vi "Write ITX.vi"(6 "Commands":string, 8 "error in":errorcluster, 9 "Notes":string, 10 "Data (Dictionary)":T1[](array[typedef]), 11 "filename":path) -> (0 "error out":errorcluster, 3 "file":path)   [LabVIEW 2020, in "Data.ITX.lvclass"]
uses:
  Data.ITX.lvclass
  Data/Typedefs/Dictionary--cluster.ctl
  Data/Data.lvclass
panel:
  out "String":string
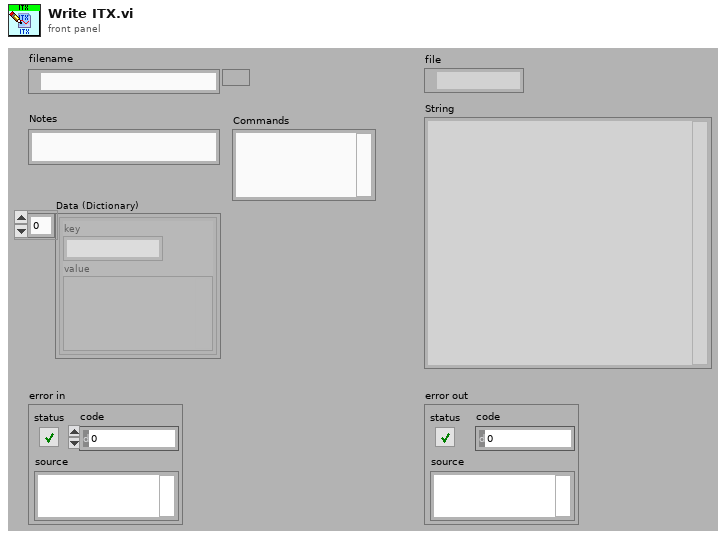
[diagram p1: front panel]
types:
  T1 = typedef "Data.lvclass/Dictionary--cluster.ctl" = cluster{"key":string, "value":variant}
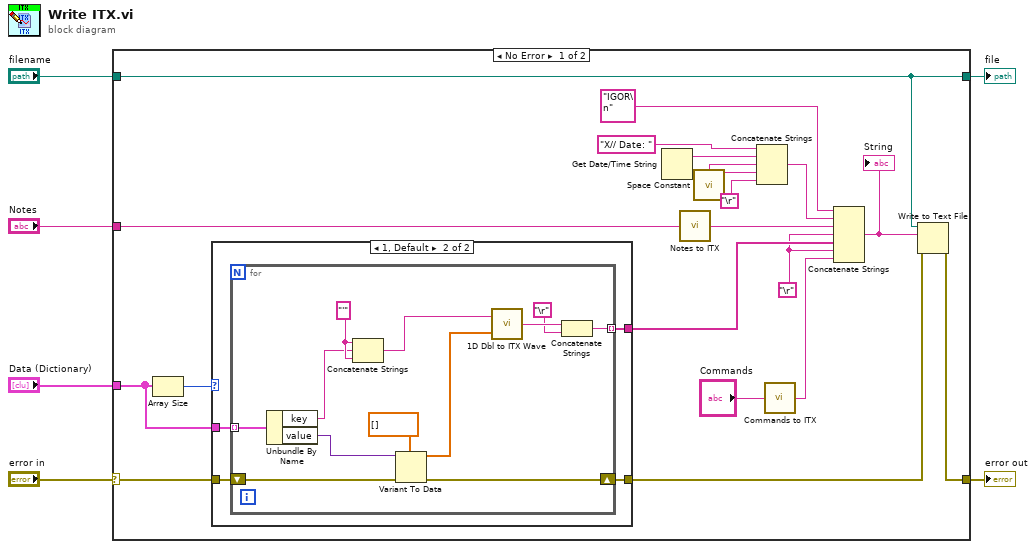
[diagram p0: block diagram]
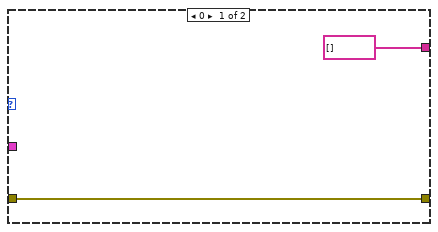
[diagram p2: hidden frame]
diagram:
  n1 = case shown="No Error" "error in" {
    selector: "error in" -> [w8 w45]
    tunnel: "filename" -> [w9 w46]
    tunnel: "Notes" -> [w19 _]
    tunnel: [w13 w45] -> w4
    tunnel: "Data (Dictionary)" -> [w10 _]
    tunnel: [w9 w46] -> w2
    frame No Error {
      w18 = "\r"
      n2 = Array Size(array=w10) -> (size(s)=w12:i32)
      n3 = case shown="1, Default" w12 {
        tunnel: [string[] [] w32] -> w21
        tunnel: w10 -> [_ w31]
        tunnel: w8 -> [w27 w30]
        tunnel: [w27 w29] -> w11
        frame 0 {
        }
        frame 1, Default {
          n4 = for {
            tunnel: [w44] -> w32 mode=indexing
            tunnel: w31 -> [w39] mode=indexing
            shift-right: [w34] -> w29
            shift-left: w30 -> [w35]
            w41 = "'"
            n5 = Unbundle By Name(w39) -> ("key"=w33:string, "value"=w37:variant)
            n6 = Concatenate Strings(w41, w33, w41) -> (w40:string)
            n7 = Variant To Data(error in=w35, type=dbl[] [] ("Data"), Variant=w37) -> (data=w36:dbl[], error out=w34:errorcluster)
            n8 = call "1D Dbl to ITX Wave.vi"("1D Array"=w36, "Wavename"=w40) -> ("ITX Wave"=w43:string)
            n9 = Concatenate Strings(w43, "\r") -> (w44:string)
          }
        }
      }
      n10 = Get Date/Time String() -> (date string=w25:string, time string=w26:string)  [unwired: 3 out]
      n11 = call "Notes to ITX.vi"("Notes"=w19) -> ("ITX Notes"=w15:string)
      n12 = call <vilib>:"Space Constant.vi"() -> ("String"=w23:string)
      n13 = Concatenate Strings("X// Date: " ("format string"), w25, w23, w26, "\r") -> (w17:string)
      n14 = call "Commands to ITX.vi"("Commands"="Commands") -> ("ITX Commands"=w14:string)
      n15 = Concatenate Strings("IGOR\n", w17, w15, w18, w21, w18, w14) -> (w20:string)
      "String" <- w20
      n16 = Write to Text File(file (use dialog)=w9, text=w20, error in=w11) -> (error out=w13:errorcluster)  [unwired: 3 out]
    }
    frame Error {
    }
  }
  "file" <- w2
  "error out" <- w4
